vi "TestTrigger.vi"() -> ()   [LabVIEW 2014]
uses:
  TriggerChannel.ctl
  <vilib>/userdefined/High Color/nirio_resource_hc.ctl
  <vilib>/FPGAPlugInAG/PCI-7813R/niLvFpga_Open_PCI-7813R.vi
  <vilib>/Utility/error.llb/Error Cluster From Error Code.vi
  <vilib>/rvi/errors/niLvFpgaAdjustHostInterfaceError.vi
  <vilib>/rvi/interface/nirviOpenFPGA/nirviOpenFPGA.xnode
  BLV/FPGA Bitfiles/W7XBolo_FPGATarget_fmain2014_oOwO-XGYwcQ.lvbitx
  BLV/f_main_2014.vi
  <vilib>/rvi/interface/nirviReadWriteControl/nirviReadWriteControl.xnode
  NiFpgaLv.dll
panel:
  out "C3DIGIN":bool
  out "C2DIGIN":bool
  out "C1DIGIN":bool
  out "C0DIGIN":bool
  out "error out":errorcluster
  in  "Trigger default: board0 (t = 0)":T1=enum."board1 (t = -1min)"
  out "Numeric":i32
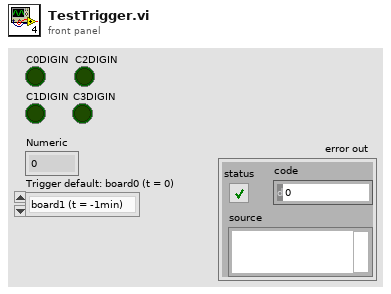
[diagram p1: front panel]
types:
  T1 = typedef "TriggerChannel.ctl" = enum16{"board0 (t = 0)", "board1 (t = -1min)", "board2 (t = -10sec)"}
  T2 = typedef "nirio_resource_hc.ctl" = tag
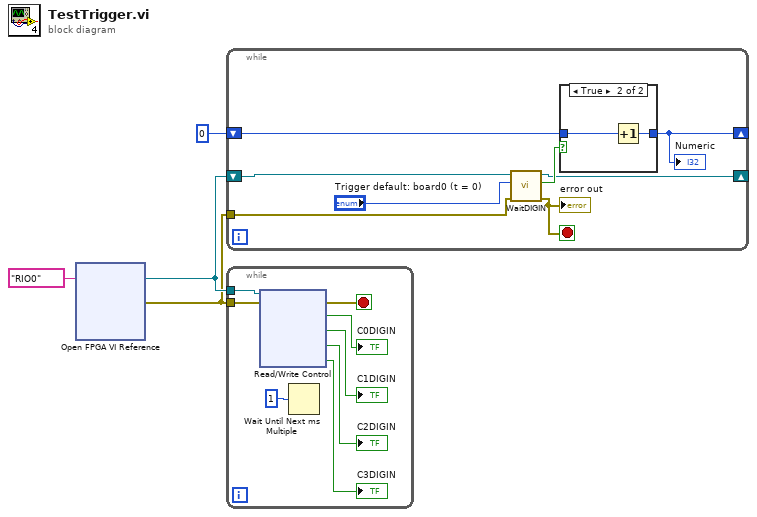
[diagram p0: block diagram]
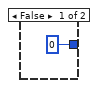
[diagram p2: hidden frame]
diagram:
  n1 = xnode "Open FPGA VI Reference"("resource name"=T2 "RIO0") -> ("FPGA VI Reference Out"=w2:refnum<k20>, "error out"=w1:errorcluster)  [unwired: 1 in]
  n2 = while {
    tunnel: w1 -> [w11]
    shift-right: [w6] -> _
    shift-left: 0 -> [w8]
    shift-right: [w7] -> _
    shift-left: w2 -> [w12]
    stop <- w10 stop-if-true
    n3 = call "WaitDIGIN.vi"("error in (no error)"=w11, "Trigger default: board0 (t = 0)"="Trigger default: board0 (t = 0)", "FPGA VI Reference In"=w12) -> ("error out"=w10:errorcluster, "TriggerFired?"=w9:bool, "FPGA VI Reference Out"=w7:refnum<k20>)  [unwired: 5 in, 1 out]
    "error out" <- w10
    n4 = case shown="True" w9 {
      tunnel: [0 w14] -> w6
      tunnel: w8 -> [_ w15]
      frame False {
      }
      frame True {
        n5 = Increment(x=w15) -> (x+1=w14:i32)
      }
    }
    "Numeric" <- w6
  }
  n6 = while {
    tunnel: w2 -> [w23]
    tunnel: w1 -> [w22]
    stop <- w21 stop-if-true
    n7 = xnode "Read/Write Control"("FPGA VI Reference In"=w23, "error in"=w22) -> ("error out"=w21:errorcluster, "C0DIGIN"=→"C0DIGIN":bool, "C1DIGIN"=→"C1DIGIN":bool, "C2DIGIN"=→"C2DIGIN":bool, "C3DIGIN"=→"C3DIGIN":bool)  [unwired: 1 out]
    n8 = Wait Until Next ms Multiple(millisecond multiple=u32 1) -> ()  [unwired: 1 out]
  }
